vi "SECoP-Exit.vi"(8 "error in (no error)":errorcluster, 11 "DLL path (in)":T1) -> (0 "error out":errorcluster)   [LabVIEW 2023, in "SECoP.lvlib"]
doc: "Call <b>\"SECoP-Exit.vi\"</b> as one of the last steps to clean things up. This will allow to unload the used external libraries.\n\n<b>DLL path</b> input of cluster from \"SECoP-Initialize.vi\""
uses:
  SECoP.lvlib
  SECoP-libraries.ctl
  SECoP-data/SECoP-data.ctl
  SECoP-error.ctl
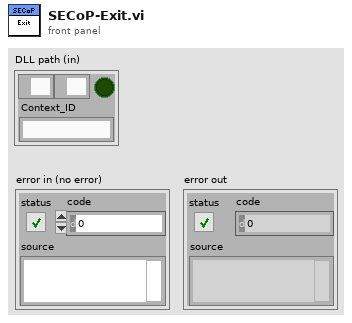
[diagram p1: front panel]
types:
  T1 = typedef "SECoP.lvlib/SECoP-libraries.ctl" = cluster{"serverDLL":path, "variantDLL":path, "cleanup_mode":bool, "Context_ID":string}
  T2 = typedef "SECoP.lvlib/SECoP-error.ctl" = i32
  T3 = typedef "SECoP.lvlib/SECoP-data.ctl" = cluster{"ptr32":u32, "ptr64":u64}
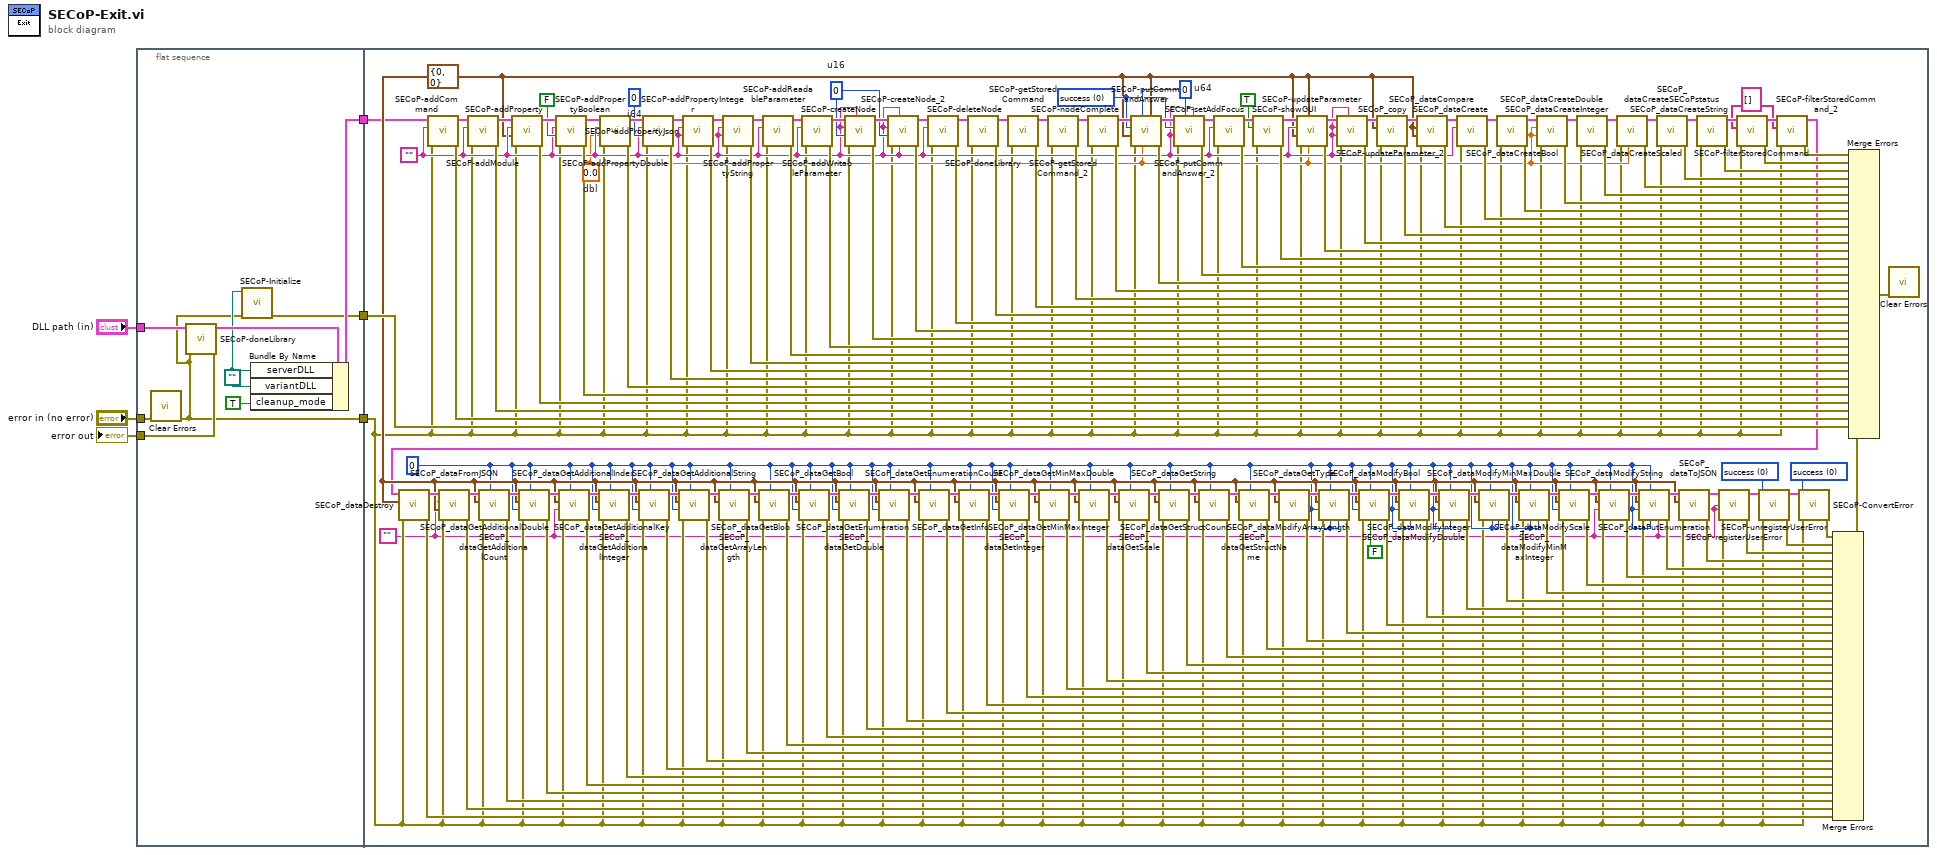
[diagram p0: block diagram]
diagram:
  n1 = flat-sequence {
    tunnel: [w8] -> w3
    tunnel: [w13] -> w4
    tunnel: "error in (no error)" -> [w14]
    tunnel: "DLL path (in)" -> [w15]
    tunnel: [w10] -> w2
    tunnel: [w7] -> w1
    tunnel: w3 -> [w19]
    tunnel: w2 -> [w28]
    tunnel: w1 -> [w169]
    frame #0 {
      w9 = path ""
      n2 = call <vilib>:"Clear Errors.vi"("error in (no error)"=w14) -> ("error out"=w8:errorcluster)  [unwired: 5 in, 1 out]
      n3 = call "SECoP-doneLibrary.vi"("error in (no error)"=w8, "DLL path (in)"=w15) -> ("error out"=w13:errorcluster, "DLL path (out)"=w11:T1)  [unwired: 8 in]
      n4 = call "SECoP-Initialize.vi"("error in (no error)"=w8, "DLL path (in)"=w9) -> ("error out"=w7:errorcluster)  [unwired: 8 in, 1 out]
      n5 = Bundle By Name(cluster=w11, "serverDLL"=w9, "variantDLL"=w9, "cleanup_mode"=TRUE) -> (w10:T1)
    }
    frame #1 {
      w16 = 0 items=["warn: missing properties"=4, "warn: buffer too small"=3, "warn: custom property"=2, "warn: no description"=1, "success"=0, "error: unknown command"=-1, "error: invalid name"=-2, "error: invalid node"=-3, "error: invalid module"=-4, "error: invalid parameter"=-5, "error: invalid property"=-6, "error: invalid command"=-7, "error: not implemented"=-8, "error: readonly"=-9, "error: no data"=-10, "error: no memory"=-11, "error: not initialized"=-12, "error: invalid value"=-13, "error: missing mandatory prop"=-14, "error: no setter/getter"=-15, "error: no setter"=-16, "error: no getter"=-17, "error: name already in use"=-18] ("SECoP error")
      w17 = T2 0 items=["warn: missing properties"=4, "warn: buffer too small"=3, "warn: custom property"=2, "warn: no description"=1, "success"=0, "error: unknown command"=-1, "error: invalid name"=-2, "error: invalid node"=-3, "error: invalid module"=-4, "error: invalid parameter"=-5, "error: invalid property"=-6, "error: invalid command"=-7, "error: not implemented"=-8, "error: readonly"=-9, "error: no data"=-10, "error: no memory"=-11, "error: not initialized"=-12, "error: invalid value"=-13, "error: missing mandatory prop"=-14, "error: no setter/getter"=-15, "error: no setter"=-16, "error: no getter"=-17, "error: name already in use"=-18] ("registered SECoP error")
      w23 = string[] [] ("filter accessibles")
      w18 = ""
      w29 = u32 0 ("Position")
      w31 = T3 {"ptr32"=0, "ptr64"=0} ("property value (SECoP_dataPtr)")
      w119 = i64 0  # i64
      w116 = 0 items=["warn: missing properties"=4, "warn: buffer too small"=3, "warn: custom property"=2, "warn: no description"=1, "success"=0, "error: unknown command"=-1, "error: invalid name"=-2, "error: invalid node"=-3, "error: invalid module"=-4, "error: invalid parameter"=-5, "error: invalid property"=-6, "error: invalid command"=-7, "error: not implemented"=-8, "error: readonly"=-9, "error: no data"=-10, "error: no memory"=-11, "error: not initialized"=-12, "error: invalid value"=-13, "error: missing mandatory prop"=-14, "error: no setter/getter"=-15, "error: no setter"=-16, "error: no getter"=-17, "error: name already in use"=-18] ("SECoP error")
      w96 = 0.0  # dbl
      w117 = u64 0  # u64
      w118 = u16 0  # u16
      w97 = ""
      n6 = call "SECoP-addCommand.vi"("error in (no error)"=w19, "command name"=w97, "DLL path (in)"=w28) -> ("error out"=w145:errorcluster, "DLL path (out)"=w143:T1)  [unwired: 7 in]
      n7 = call "SECoP-addModule.vi"("error in (no error)"=w19, "module name"=w97, "DLL path (in)"=w143) -> ("error out"=w146:errorcluster, "DLL path (out)"=w142:T1)  [unwired: 7 in]
      n8 = call "SECoP-addProperty.vi"("error in (no error)"=w19, "property value (SECoP_data)"=w31, "property name"=w97, "DLL path (in)"=w142) -> ("error out"=w147:errorcluster, "DLL path (out)"=w141:T1)  [unwired: 6 in]
      n9 = call "SECoP-addPropertyBoolean.vi"("error in (no error)"=w19, "property value"=FALSE, "property name"=w97, "DLL path (in)"=w141) -> ("error out"=w148:errorcluster, "DLL path (out)"=w140:T1)  [unwired: 6 in]
      n10 = call "SECoP-addPropertyDouble.vi"("error in (no error)"=w19, "property value"=w96, "property name"=w97, "DLL path (in)"=w140) -> ("error out"=w149:errorcluster, "DLL path (out)"=w139:T1)  [unwired: 6 in]
      n11 = call "SECoP-addPropertyInteger.vi"("error in (no error)"=w19, "property value"=w119, "property name"=w97, "DLL path (in)"=w139) -> ("error out"=w150:errorcluster, "DLL path (out)"=w138:T1)  [unwired: 6 in]
      n12 = call "SECoP-addPropertyJson.vi"("error in (no error)"=w19, "property value"=w97, "property name"=w97, "DLL path (in)"=w138) -> ("error out"=w151:errorcluster, "DLL path (out)"=w137:T1)  [unwired: 6 in]
      n13 = call "SECoP-addPropertyString.vi"("error in (no error)"=w19, "property value"=w97, "property name"=w97, "DLL path (in)"=w137) -> ("error out"=w152:errorcluster, "DLL path (out)"=w136:T1)  [unwired: 6 in]
      n14 = call "SECoP-addReadableParameter.vi"("error in (no error)"=w19, "parameter name"=w97, "DLL path (in)"=w136) -> ("error out"=w153:errorcluster, "DLL path (out)"=w135:T1)  [unwired: 7 in]
      n15 = call "SECoP-addWritableParameter.vi"("error in (no error)"=w19, "parameter name"=w97, "DLL path (in)"=w135) -> ("error out"=w154:errorcluster, "DLL path (out)"=w134:T1)  [unwired: 7 in]
      n16 = call "SECoP-createNode.vi"("description"=w97, "error in (no error)"=w19, "TCP port"=w118, "node id"=w97, "DLL path (in)"=w134) -> ("error out"=w155:errorcluster, "DLL path (out)"=w133:T1)  [unwired: 5 in]
      n17 = call "SECoP-createNode_2.vi"("Interface"=w97, "description"=w97, "error in (no error)"=w19, "TCP port"=w118, "node id"=w97, "DLL path (in)"=w133) -> ("error out"=w156:errorcluster, "DLL path (out)"=w132:T1)  [unwired: 4 in]
      n18 = call "SECoP-deleteNode.vi"("error in (no error)"=w19, "node id"=w97, "DLL path (in)"=w132) -> ("error out"=w157:errorcluster, "DLL path (out)"=w131:T1)  [unwired: 7 in]
      n19 = call "SECoP-doneLibrary.vi"("error in (no error)"=w19, "DLL path (in)"=w131) -> ("error out"=w158:errorcluster, "DLL path (out)"=w130:T1)  [unwired: 8 in]
      n20 = call "SECoP-getStoredCommand.vi"("error in (no error)"=w19, "DLL path (in)"=w130) -> ("error out"=w159:errorcluster, "DLL path (out)"=w128:T1)  [unwired: 4 in, 4 out]
      n21 = call "SECoP-getStoredCommand_2.vi"("error in (no error)"=w19, "DLL path (in)"=w128) -> ("error out"=w160:errorcluster, "DLL path (out)"=w27:T1)  [unwired: 4 in, 4 out]
      n22 = call "SECoP-nodeComplete.vi"("error in (no error)"=w19, "DLL path (in)"=w27) -> ("error out"=w161:errorcluster, "DLL path (out)"=w127:T1)  [unwired: 8 in]
      n23 = call "SECoP-putCommandAnswer.vi"("sigma (SECoP_data)"=w31, "timestamp"=w96, "command id"=w117, "error in (no error)"=w19, "value (SECoP_data)"=w31, "SECoP error"=w116, "DLL path (in)"=w127) -> ("error out"=w162:errorcluster, "DLL path (out)"=w126:T1)  [unwired: 3 in]
      n24 = call "SECoP-putCommandAnswer_2.vi"("sigma"=w97, "command id"=w117, "error in (no error)"=w19, "value"=w97, "SECoP error"=w116, "DLL path (in)"=w126) -> ("error out"=w163:errorcluster, "DLL path (out)"=w125:T1)  [unwired: 4 in]
      n25 = call "SECoP-setAddFocus.vi"("error in (no error)"=w19, "key name"=w97, "DLL path (in)"=w125) -> ("error out"=w164:errorcluster, "DLL path (out)"=w123:T1)  [unwired: 7 in]
      n26 = call "SECoP-showGUI.vi"("error in (no error)"=w19, "show GUI"=TRUE, "DLL path (in)"=w123) -> ("error out"=w167:errorcluster, "DLL path (out)"=w120:T1)  [unwired: 7 in]
      n27 = call "SECoP-updateParameter.vi"("Timestamp"=w96, "sigma (SECoP_data)"=w31, "error in (no error)"=w19, "value (SECoP_data)"=w31, "parameter name"=w97, "DLL path (in)"=w120) -> ("error out"=w165:errorcluster, "DLL path (out)"=w124:T1)  [unwired: 4 in]
      n28 = call "SECoP-updateParameter_2.vi"("sigma"=w97, "error in (no error)"=w19, "value"=w97, "parameter name"=w97, "DLL path (in)"=w124) -> ("error out"=w166:errorcluster, "DLL path (out)"=w115:T1)  [unwired: 5 in]
      n29 = call "SECoP_copy.vi"("error in (no error)"=w19, "SECoP_dataPtr in"=w31, "DLL path (in)"=w115) -> ("error out"=w98:errorcluster, "DLL path (out)"=w114:T1)  [unwired: 6 in, 1 out]
      n30 = call "SECoP_dataCompare.vi"("error in (no error)"=w19, "SECoP_dataPtr (2)"=w31, "SECoP_dataPtr (1)"=w31, "DLL path (in)"=w114) -> ("error out"=w99:errorcluster, "DLL path (out)"=w113:T1)  [unwired: 5 in, 1 out]
      n31 = call "SECoP_dataCreate.vi"("error in (no error)"=w19, "Description"=w97, "DLL path (in)"=w113) -> ("error out"=w100:errorcluster, "DLL path (out)"=w112:T1)  [unwired: 6 in, 1 out]
      n32 = call "SECoP_dataCreateBool.vi"("error in (no error)"=w19, "DLL path (in)"=w112) -> ("error out"=w101:errorcluster, "DLL path (out)"=w111:T1)  [unwired: 7 in, 1 out]
      n33 = call "SECoP_dataCreateDouble.vi"("error in (no error)"=w19, "maximum value"=w96, "minimum value"=w96, "DLL path (in)"=w111) -> ("error out"=w102:errorcluster, "DLL path (out)"=w110:T1)  [unwired: 5 in, 1 out]
      n34 = call "SECoP_dataCreateInteger.vi"("error in (no error)"=w19, "DLL path (in)"=w110) -> ("error out"=w103:errorcluster, "DLL path (out)"=w109:T1)  [unwired: 7 in, 1 out]
      n35 = call "SECoP_dataCreateScaled.vi"("scale factor"=w96, "error in (no error)"=w19, "DLL path (in)"=w109) -> ("error out"=w104:errorcluster, "DLL path (out)"=w108:T1)  [unwired: 6 in, 1 out]
      n36 = call "SECoP_dataCreateSECoPstatus.vi"("error in (no error)"=w19, "DLL path (in)"=w108) -> ("error out"=w105:errorcluster, "DLL path (out)"=w107:T1)  [unwired: 7 in, 1 out]
      n37 = call "SECoP_dataCreateString.vi"("error in (no error)"=w19, "DLL path (in)"=w107) -> ("error out"=w106:errorcluster, "DLL path (out)"=w26:T1)  [unwired: 7 in, 1 out]
      n38 = call "SECoP-filterStoredCommand.vi"("error in (no error)"=w19, "filter accessibles"=w23, "DLL path (in)"=w26) -> ("error out"=w170:errorcluster, "DLL path (out)"=w25:T1)  [unwired: 3 in, 4 out]
      n39 = call "SECoP-filterStoredCommand_2.vi"("error in (no error)"=w19, "filter accessibles"=w23, "DLL path (in)"=w25) -> ("error out"=w171:errorcluster, "DLL path (out)"=w24:T1)  [unwired: 3 in, 4 out]
      n40 = call "SECoP_dataDestroy.vi"("error in (no error)"=w19, "SECoP_dataPtr"=w31, "DLL path (in)"=w24) -> ("error out"=w74:errorcluster, "DLL path (out)"=w168:T1)  [unwired: 7 in]
      n41 = call "SECoP_dataFromJSON.vi"("error in (no error)"=w19, "hint: SECoP_dataPtr"=w31, "JSON"=w18, "DLL path (in)"=w168) -> ("error out"=w73:errorcluster, "DLL path (out)"=w95:T1)  [unwired: 5 in, 1 out]
      n42 = call "SECoP_dataGetAdditionalCount.vi"("Position"=w29, "error in (no error)"=w19, "SECoP_dataPtr"=w31, "DLL path (in)"=w95) -> ("error out"=w72:errorcluster, "DLL path (out)"=w94:T1)  [unwired: 5 in, 1 out]
      n43 = call "SECoP_dataGetAdditionalDouble.vi"("Position"=w29, "error in (no error)"=w19, "Index"=w29, "SECoP_dataPtr"=w31, "DLL path (in)"=w94) -> ("error out"=w71:errorcluster, "DLL path (out)"=w93:T1)  [unwired: 4 in, 1 out]
      n44 = call "SECoP_dataGetAdditionalIndex.vi"("Position"=w29, "error in (no error)"=w19, "key name"=w18, "SECoP_dataPtr"=w31, "DLL path (in)"=w93) -> ("error out"=w70:errorcluster, "DLL path (out)"=w92:T1)  [unwired: 4 in, 1 out]
      n45 = call "SECoP_dataGetAdditionalInteger.vi"("Position"=w29, "error in (no error)"=w19, "Index"=w29, "SECoP_dataPtr"=w31, "DLL path (in)"=w92) -> ("error out"=w69:errorcluster, "DLL path (out)"=w91:T1)  [unwired: 4 in, 1 out]
      n46 = call "SECoP_dataGetAdditionalKey.vi"("Position"=w29, "error in (no error)"=w19, "Index"=w29, "SECoP_dataPtr"=w31, "DLL path (in)"=w91) -> ("error out"=w68:errorcluster, "DLL path (out)"=w90:T1)  [unwired: 4 in, 1 out]
      n47 = call "SECoP_dataGetAdditionalString.vi"("Position"=w29, "error in (no error)"=w19, "Index"=w29, "SECoP_dataPtr"=w31, "DLL path (in)"=w90) -> ("error out"=w66:errorcluster, "DLL path (out)"=w89:T1)  [unwired: 4 in, 1 out]
      n48 = call "SECoP_dataGetArrayLength.vi"("Position"=w29, "error in (no error)"=w19, "SECoP_dataPtr"=w31, "DLL path (in)"=w89) -> ("error out"=w67:errorcluster, "DLL path (out)"=w88:T1)  [unwired: 3 in, 3 out]
      n49 = call "SECoP_dataGetBlob.vi"("Position"=w29, "error in (no error)"=w19, "SECoP_dataPtr in"=w31, "DLL path (in)"=w88) -> ("error out"=w65:errorcluster, "DLL path (out)"=w87:T1)  [unwired: 5 in, 1 out]
      n50 = call "SECoP_dataGetBool.vi"("Position"=w29, "error in (no error)"=w19, "Index"=w29, "SECoP_dataPtr"=w31, "DLL path (in)"=w87) -> ("error out"=w64:errorcluster, "DLL path (out)"=w86:T1)  [unwired: 4 in, 1 out]
      n51 = call "SECoP_dataGetDouble.vi"("Position"=w29, "error in (no error)"=w19, "Index"=w29, "SECoP_dataPtr"=w31, "DLL path (in)"=w86) -> ("error out"=w63:errorcluster, "DLL path (out)"=w85:T1)  [unwired: 4 in, 1 out]
      n52 = call "SECoP_dataGetEnumeration.vi"("Position"=w29, "error in (no error)"=w19, "Index"=w29, "SECoP_dataPtr in"=w31, "DLL path (in)"=w85) -> ("error out"=w62:errorcluster, "DLL path (out)"=w84:T1)  [unwired: 3 in, 2 out]
      n53 = call "SECoP_dataGetEnumerationCount.vi"("Position"=w29, "error in (no error)"=w19, "SECoP_dataPtr"=w31, "DLL path (in)"=w84) -> ("error out"=w61:errorcluster, "DLL path (out)"=w83:T1)  [unwired: 5 in, 1 out]
      n54 = call "SECoP_dataGetInfo.vi"("Position"=w29, "error in (no error)"=w19, "SECoP_dataPtr"=w31, "DLL path (in)"=w83) -> ("error out"=w60:errorcluster, "DLL path (out)"=w82:T1)  [unwired: 3 in, 3 out]
      n55 = call "SECoP_dataGetInteger.vi"("Position"=w29, "error in (no error)"=w19, "Index"=w29, "SECoP_dataPtr"=w31, "DLL path (in)"=w82) -> ("error out"=w59:errorcluster, "DLL path (out)"=w81:T1)  [unwired: 4 in, 1 out]
      n56 = call "SECoP_dataGetMinMaxDouble.vi"("Position"=w29, "error in (no error)"=w19, "SECoP_dataPtr"=w31, "DLL path (in)"=w81) -> ("error out"=w58:errorcluster, "DLL path (out)"=w80:T1)  [unwired: 4 in, 2 out]
      n57 = call "SECoP_dataGetMinMaxInteger.vi"("Position"=w29, "error in (no error)"=w19, "SECoP_dataPtr"=w31, "DLL path (in)"=w80) -> ("error out"=w56:errorcluster, "DLL path (out)"=w79:T1)  [unwired: 4 in, 2 out]
      n58 = call "SECoP_dataGetScale.vi"("Position"=w29, "error in (no error)"=w19, "SECoP_dataPtr"=w31, "DLL path (in)"=w79) -> ("error out"=w57:errorcluster, "DLL path (out)"=w78:T1)  [unwired: 5 in, 1 out]
      n59 = call "SECoP_dataGetString.vi"("Position"=w29, "error in (no error)"=w19, "SECoP_dataPtr"=w31, "DLL path (in)"=w78) -> ("error out"=w55:errorcluster, "DLL path (out)"=w77:T1)  [unwired: 5 in, 1 out]
      n60 = call "SECoP_dataGetStructCount.vi"("Position"=w29, "error in (no error)"=w19, "SECoP_dataPtr"=w31, "DLL path (in)"=w77) -> ("error out"=w54:errorcluster, "DLL path (out)"=w76:T1)  [unwired: 5 in, 1 out]
      n61 = call "SECoP_dataGetStructName.vi"("Position"=w29, "error in (no error)"=w19, "SECoP_dataPtr in"=w31, "DLL path (in)"=w76) -> ("error out"=w53:errorcluster, "DLL path (out)"=w75:T1)  [unwired: 5 in, 1 out]
      n62 = call "SECoP_dataGetType.vi"("error in (no error)"=w19, "SECoP_dataPtr"=w31, "DLL path (in)"=w75) -> ("error out"=w52:errorcluster, "DLL path (out)"=w48:T1)  [unwired: 6 in, 1 out]
      n63 = call "SECoP_dataModifyArrayLength.vi"("maximum length"=w29, "minimum length"=w29, "Position"=w29, "error in (no error)"=w19, "array length"=w29, "SECoP_dataPtr"=w31, "DLL path (in)"=w48) -> ("error out"=w51:errorcluster, "DLL path (out)"=w47:T1)  [unwired: 3 in]
      n64 = call "SECoP_dataModifyBool.vi"("Value"=FALSE, "Position"=w29, "error in (no error)"=w19, "Index"=w29, "SECoP_dataPtr"=w31, "DLL path (in)"=w47) -> ("error out"=w50:errorcluster, "DLL path (out)"=w46:T1)  [unwired: 4 in]
      n65 = call "SECoP_dataModifyDouble.vi"("Value"=w29, "Position"=w29, "error in (no error)"=w19, "Index"=w29, "SECoP_data"=w31, "DLL path (in)"=w46) -> ("error out"=w49:errorcluster, "DLL path (out)"=w45:T1)  [unwired: 4 in]
      n66 = call "SECoP_dataModifyInteger.vi"("Value"=w29, "Position"=w29, "error in (no error)"=w19, "Index"=w29, "SECoP_data"=w31, "DLL path (in)"=w45) -> ("error out"=w38:errorcluster, "DLL path (out)"=w44:T1)  [unwired: 4 in]
      n67 = call "SECoP_dataModifyMinMaxDouble.vi"("maximum value"=w29, "minimum value"=w29, "Position"=w29, "error in (no error)"=w19, "SECoP_dataPtr"=w31, "DLL path (in)"=w44) -> ("error out"=w37:errorcluster, "DLL path (out)"=w43:T1)  [unwired: 4 in]
      n68 = call "SECoP_dataModifyMinMaxInteger.vi"("maximum value"=w29, "minimum value"=w29, "Position"=w29, "error in (no error)"=w19, "SECoP_dataPtr"=w31, "DLL path (in)"=w43) -> ("error out"=w36:errorcluster, "DLL path (out)"=w42:T1)  [unwired: 4 in]
      n69 = call "SECoP_dataModifyScale.vi"("Position"=w29, "error in (no error)"=w19, "scale factor"=w29, "SECoP_dataPtr"=w31, "DLL path (in)"=w42) -> ("error out"=w35:errorcluster, "DLL path (out)"=w41:T1)  [unwired: 5 in]
      n70 = call "SECoP_dataModifyString.vi"("Position"=w29, "error in (no error)"=w19, "Value"=w18, "SECoP_dataPtr"=w31, "DLL path (in)"=w41) -> ("error out"=w34:errorcluster, "DLL path (out)"=w40:T1)  [unwired: 5 in]
      n71 = call "SECoP_dataPutEnumeration.vi"("enumeration_name"=w18, "Enumval"=w29, "Position"=w29, "error in (no error)"=w19, "Index"=w29, "SECoP_dataPtr in"=w31, "DLL path (in)"=w40) -> ("error out"=w33:errorcluster, "DLL path (out)"=w39:T1)  [unwired: 3 in]
      n72 = call "SECoP_dataToJSON.vi"("error in (no error)"=w19, "SECoP_dataPtr"=w31, "DLL path (in)"=w39) -> ("error out"=w32:errorcluster, "DLL path (out)"=w22:T1)  [unwired: 6 in, 1 out]
      n73 = call "SECoP-registerUserError.vi"("error in (no error)"=w19, "message text"=w18, "SECoP-Error"=w18, "DLL path (in)"=w22) -> ("error out"=w172:errorcluster, "DLL path (out)"=w21:T1)  [unwired: 5 in, 1 out]
      n74 = call "SECoP-unregisterUserError.vi"("error in (no error)"=w19, "registered SECoP error"=w17, "DLL path (in)"=w21) -> ("error out"=w173:errorcluster, "DLL path (out)"=w20:T1)  [unwired: 7 in]
      n75 = call "SECoP-ConvertError.vi"("return code"=w16, "error in (no error)"=w19, "DLL path (in)"=w20) -> ("error out"=w174:errorcluster)  [unwired: 7 in, 1 out]
      n76 = Merge Errors(w174, w173, w172, w32, w33, w34, w35, w36, w37, w38, w49, w50, w51, w52, w53, w54, w55, w57, w56, w58, w59, w60, w61, w62, w63, w64, w65, w67, w66, w68, w69, w70, w71, w72, w73, w74) -> (w144:errorcluster)
      n77 = Merge Errors(w171, w170, w106, w105, w104, w103, w102, w101, w100, w99, w98, w166, w165, w167, w164, w163, w162, w161, w160, w159, w158, w157, w156, w155, w154, w153, w152, w151, w150, w149, w148, w147, w146, w145, w169, w144) -> (w121:errorcluster)
      n78 = call <vilib>:"Clear Errors.vi"("error in (no error)"=w121) -> ()  [unwired: 5 in, 2 out]
    }
  }
  "error out" <- w4
